vi "ForecastData Long.vi"(8 "error in":errorcluster, 10 "ForecastData":T1, 11 "SCADA in":refnum<class "EMS.lvclass">) -> (0 "error out":errorcluster, 3 "SCADA out":refnum<class "EMS.lvclass">)   [LabVIEW 2018, in "EMS Core.lvlib" / "EMS.lvclass"]
uses:
  EMS.lvclass
  <vilib>/ORNL/CSEISMIC DDS/CSEISMIC DDS Base/Data Types/ForecastData_Data.ctl
  <vilib>/ORNL/CSEISMIC DDS/CSEISMIC DDS Base/Data Types/Controls/DeviceID.ctl
  EMS.lvclass/EMS.ctl
  IED Actors/ForecastData Actor/ForecastData Messages/Write ForecastData_Long Msg/Write ForecastData_Long Msg.lvclass/Write ForecastData_Long Msg.ctl
  <vilib>/ActorFramework/Message Enqueuer/Message Enqueuer.lvclass/Message Enqueuer.ctl
  <vilib>/ActorFramework/Message Enqueuer/Enqueue.vi
  IED Actors/ForecastData Actor/ForecastData Messages/Write ForecastData_Long Msg/Write ForecastData_Long Msg.lvclass
  C:/Program Files (x86)/National Instruments/LabVIEW 2018/vi.lib/ActorFramework/Message/Message.lvclass
  <vilib>/ActorFramework/Message Priority Queue/Priority Enqueue.vi
  <vilib>/ORNL/CSEISMIC DDS/CSEISMIC DDS Base/CSEISMIC DDS.lvclass
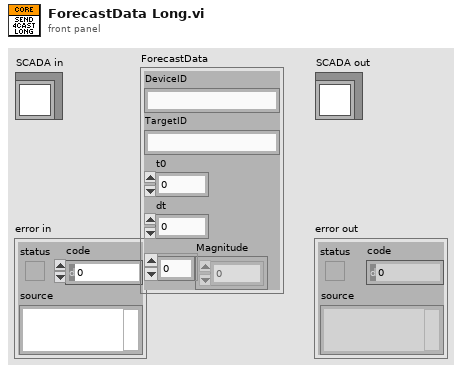
[diagram p1: front panel]
types:
  T1 = typedef "CSEISMIC DDS.lvlib/CSEISMIC DDS.lvclass/ForecastData_Data.ctl" = cluster{"DeviceID":T2, "TargetID":T2, "t0":dbl, "dt":dbl, "Magnitude":dbl[]}
  T2 = typedef "CSEISMIC DDS.lvlib/CSEISMIC DDS.lvclass/DeviceID.ctl" = string
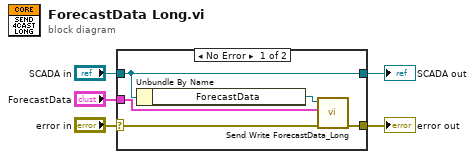
[diagram p0: block diagram]
diagram:
  n1 = case shown="No Error" "error in" {
    selector: "error in" -> [w8 w12]
    tunnel: [w7 w12] -> w4
    tunnel: [w9 w11] -> w2
    tunnel: "SCADA in" -> [w9 w11]
    tunnel: "ForecastData" -> [w6 _]
    frame No Error {
      n2 = Unbundle By Name(w9) -> ("ForecastData"=w10:refnum<class "Message Enqueuer.lvclass">)
      n3 = call "Send Write ForecastData_Long.vi"("error in (no error)"=w8, "ForecastData"=w6, "Message Enqueuer"=w10) -> ("error out"=w7:errorcluster)  [unwired: 7 in, 1 out]
    }
    frame Error {
    }
  }
  "error out" <- w4
  "SCADA out" <- w2
